vi "Particle Analysis Example.vi"() -> ()   [LabVIEW 2011]
doc: "This example performs a series of grayscale filtering, threshold, binary morphology, and particle analysis operations to measure the areas of all the large circular particles of the image."
uses:
  <vilib>/vision/NI_Vision_Development_Module.lvlib
panel:
  out "Source Image":T1(plugin-control) caption="Rejected Border"
  in  "Font, Size & Style":T2={"Desired Font (Application)"=enum."Application Font", "[User-specified Font]"={"Font Name"="", "Size"=12, "Strikeout?"=FALSE, "Italic?"=FALSE, "Underline?"=FALSE, "Outline?"=FALSE, "Shadow?"=FALSE, "Bold?"=FALSE, "Rotation Angle"=0.0}, "Horizontal Alignment"=0, "Vertical Alignment"=0} {"Vertical Alignment" items=["Bottom", "Top", "Baseline"]; "Horizontal Alignment" items=["Left", "Center", "Right"]; "[User-specified Font]"."Rotation Angle" format="%.2f"}
  in  "Stop":bool
  in  "Run Current Step":bool
  out "Blob Analysis Steps":i32(listbox)
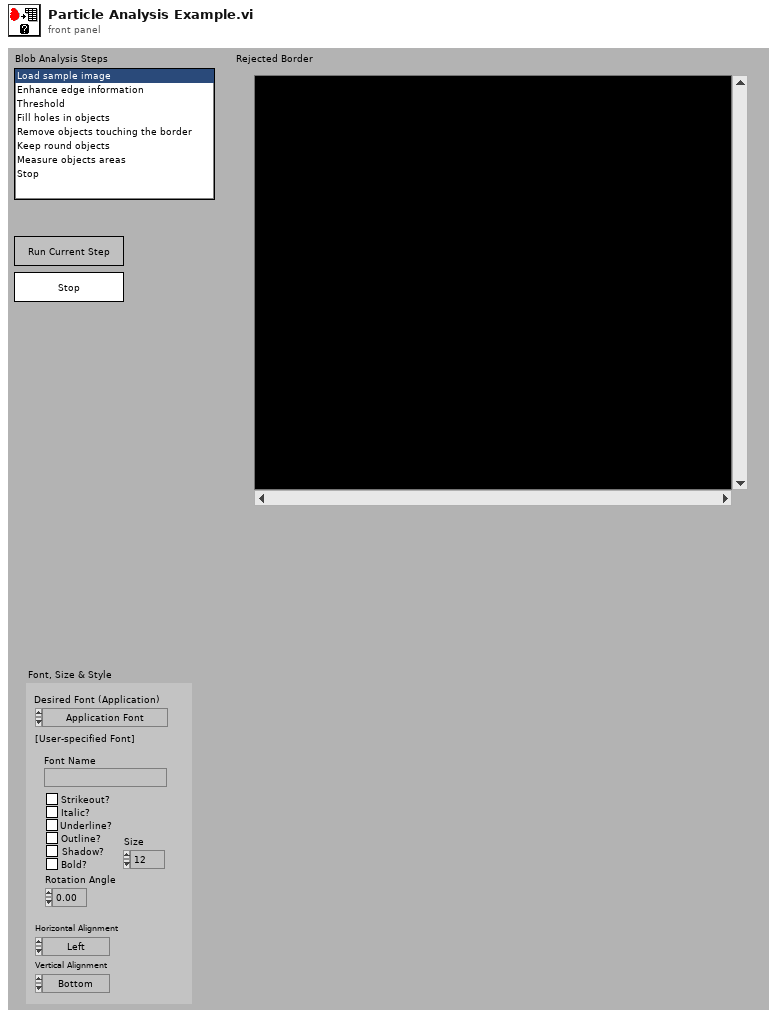
[diagram p1: front panel]
types:
  T1 = typedef "IMAQ Image.ctl" = refnum<image>
  T2 = cluster{"Desired Font (Application)":enum16{"User-specified Font", "Application Font", "System Font", "Dialog Font"}, "[User-specified Font]":cluster{"Font Name":string, "Size":i16, "Strikeout?":bool, "Italic?":bool, "Underline?":bool, "Outline?":bool, "Shadow?":bool, "Bold?":bool, "Rotation Angle":dbl}, "Horizontal Alignment":i16, "Vertical Alignment":i16}
  T3 = enum32{"", "Gradient", "Laplacian", "Smoothing", "Gaussian"}
  T4 = typedef "Particle Parameters" = i32
  T5 = cluster{"Measurement Parameter":T4, "Range Lower Value":dbl, "Range Upper Value":dbl, "Range":bool, "Measurement Type":bool}[]
  T6 = cluster{"Particle Measurements (Pixels)[0]":dbl, "Particle Measurements (Pixels)[1]":dbl, "Particle Measurements (Pixels)[2]":dbl}
  T7 = cluster{"Particle Measurements (Pixels)[0]":dbl, "Particle Measurements (Pixels)[1]":dbl}
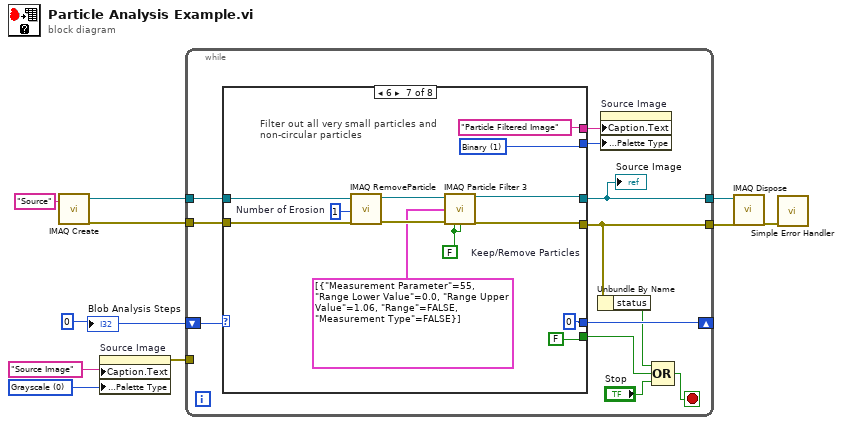
[diagram p0: block diagram]
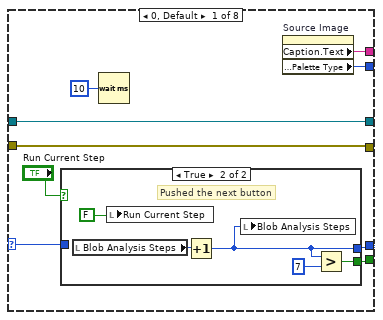
[diagram p2: hidden frame]
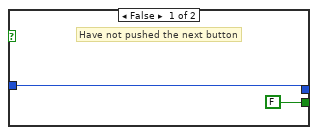
[diagram p3: hidden frame]
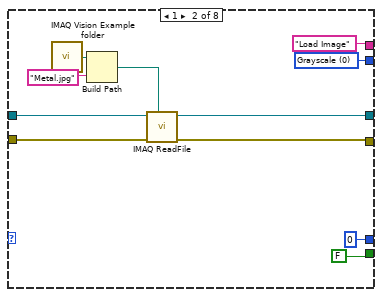
[diagram p4: hidden frame]
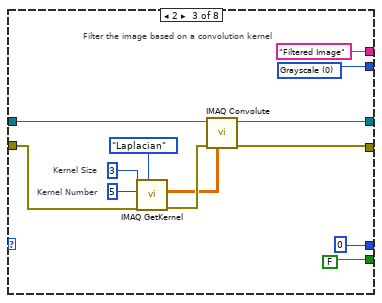
[diagram p5: hidden frame]
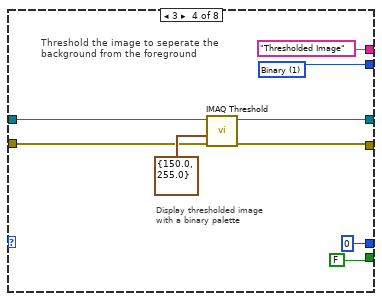
[diagram p6: hidden frame]
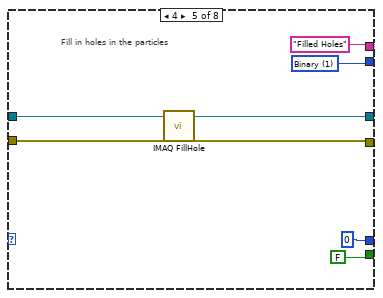
[diagram p7: hidden frame]
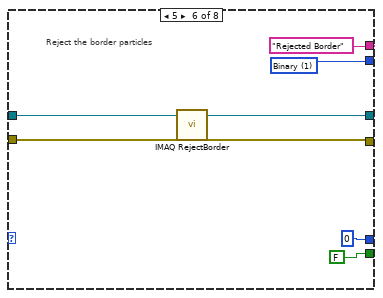
[diagram p8: hidden frame]
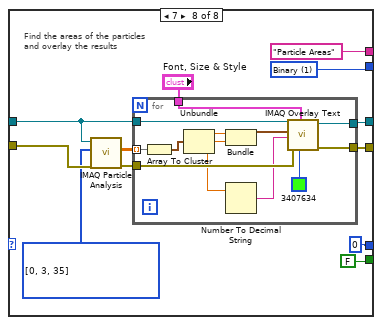
[diagram p9: hidden frame]
diagram:
  w6 = 0
  w7 = u32 0 items=["Grayscale", "Binary", "Gradient", "Rainbow", "Temperature", "User Defined"] ("Palette:Palette Type")
  n1 = call "IMAQ Create"("Image Name"="Source") -> ("New Image"=w2:T1, "error out"=w1:errorcluster)  [unwired: 3 in, 1 out]
  n2 = property on="Source Image" class="ImageControl"("Caption.Text"="Source Image", "Palette:Palette Type"=w7) -> (error out=w9:errorcluster)  [unwired: 2 in, 1 out]
  n3 = while {
    tunnel: w2 -> [w22]
    tunnel: w1 -> [w21]
    shift-right: [w17] -> _
    shift-left: w6 -> [w18]
    tunnel: w9 -> [_]
    tunnel: [w12] -> w5
    tunnel: [w11] -> w4
    stop <- w20 stop-if-true
    n4 = case shown="6" w18 {
      selector: w18 -> [w30 _ _ _ _ _ _ _]
      tunnel: w22 -> [w28 w47 w57 w70 w79 w87 w97 w111]
      tunnel: w21 -> [w29 w46 w51 w63 w73 w81 w91 w103]
      tunnel: [w29 w44 w55 w66 w76 w84 w95 w107] -> w12
      tunnel: [w23 0 0 0 0 0 0 0] -> w17
      tunnel: [w28 w45 w54 w68 w75 w83 w93 w108] -> w11
      tunnel: [w27 "Load Image" ("Title") "Filtered Image" ("Title") "Thresholded Image" ("Title") "Filled Holes" ("Title") "Rejected Border" ("Title") "Particle Filtered Image" ("Title") "Particle Areas" ("Title")] -> w15
      tunnel: [w26 w40 w50 w64 w72 w80 w90 w105] -> w16
      tunnel: [w25 FALSE FALSE FALSE FALSE FALSE FALSE FALSE] -> w13
      frame 0, Default {
        n5 = case shown="True" "Run Current Step" {
          tunnel: w30 -> [w32 _]
          tunnel: [FALSE w35] -> w25
          tunnel: [w32 w34] -> w23
          frame False {
            # "Have not pushed the next button"
          }
          frame True {
            # "Pushed the next button"
            n6 = local read "Blob Analysis Steps"() -> (w37:i32)
            n7 = local write "Run Current Step"(FALSE) -> ()
            n8 = Increment(x=w37) -> (x+1=w34:i32)
            n9 = local write "Blob Analysis Steps"(w34) -> ()
            n10 = Greater?(x=w34, y=7) -> (0:w35:bool)
          }
        }
        n11 = Wait (ms)(milliseconds to wait=u32 10) -> ()  [unwired: 1 out]
        n12 = property on="Source Image" class="ImageControl"() -> ("Caption.Text"=w27:string, "Palette:Palette Type"=w26:u32)  [unwired: 2 in, 2 out]
      }
      frame 1 {
        w40 = u32 0 items=["Grayscale", "Binary", "Gradient", "Rainbow", "Temperature", "User Defined"] ("Palette:Palette Type")
        n13 = call "IMAQ Vision Example folder.vi"() -> ("Example Image Path"=w48:path)  [unwired: 1 out]
        n14 = Build Path(base path=w48, name or relative path="Metal.jpg") -> (appended path=w43:path)
        n15 = call "IMAQ ReadFile"("File Path"=w43, "error in (no error)"=w46, "Image"=w47) -> ("error out"=w44:errorcluster, "Image Out"=w45:T1)  [unwired: 2 in, 5 out]
      }
      frame 2 {
        w50 = u32 0 items=["Grayscale", "Binary", "Gradient", "Rainbow", "Temperature", "User Defined"] ("Palette:Palette Type")
        # "Kernel Number"
        # "Kernel Size"
        # "Filter the image based on a convolution kernel"
        n16 = call "IMAQ GetKernel"("Kernel Family"=T3."Laplacian", "error in (no error)"=w51, "Kernel Number"=5, "Kernel Size (3,5,...)"=3) -> ("error out"=w62:errorcluster, "Kernel"=w61:sgl[][])  [unwired: 1 in, 5 out]
        n17 = call "IMAQ Convolute"("Kernel"=w61, "error in (no error)"=w62, "Image Src"=w57) -> ("error out"=w55:errorcluster, "Image Dst Out"=w54:T1)  [unwired: 4 in, 3 out]
      }
      frame 3 {
        w64 = u32 1 items=["Grayscale", "Binary", "Gradient", "Rainbow", "Temperature", "User Defined"] ("Palette:Palette Type")
        # "Display thresholded image with a binary palette"
        # "Threshold the image to seperate the background from the foreground"
        n18 = call "IMAQ Threshold"("error in (no error)"=w63, "Range"=cluster{"Lower value":sgl, "Upper value":sgl} {"Lower value"=150.0, "Upper value"=255.0}, "Image Src"=w70) -> ("error out"=w66:errorcluster, "Image Dst Out"=w68:T1)  [unwired: 3 in, 4 out]
      }
      frame 4 {
        w72 = u32 1 items=["Grayscale", "Binary", "Gradient", "Rainbow", "Temperature", "User Defined"] ("Palette:Palette Type")
        # "Fill in holes in the particles"
        n19 = call "IMAQ FillHole"("error in (no error)"=w73, "Image Src"=w79) -> ("error out"=w76:errorcluster, "Image Dst Out"=w75:T1)  [unwired: 2 in, 2 out]
      }
      frame 5 {
        w80 = u32 1 items=["Grayscale", "Binary", "Gradient", "Rainbow", "Temperature", "User Defined"] ("Palette:Palette Type")
        # "Reject the border particles"
        n20 = call "IMAQ RejectBorder"("error in (no error)"=w81, "Image Src"=w87) -> ("error out"=w84:errorcluster, "Image Dst Out"=w83:T1)  [unwired: 2 in, 2 out]
      }
      frame 6 {
        w90 = u32 1 items=["Grayscale", "Binary", "Gradient", "Rainbow", "Temperature", "User Defined"] ("Palette:Palette Type")
        w98 = 1  # Number of Erosion
        w88 = FALSE  # Keep/Remove Particles
        # "Filter out all very small particles and non-circular particles"
        n21 = call "IMAQ RemoveParticle"("error in (no error)"=w91, "Number of Erosion"=w98, "Image Src"=w97) -> ("error out"=w100:errorcluster, "Image Dst Out"=w99:T1)  [unwired: 4 in, 3 out]
        n22 = call "IMAQ Particle Filter 3"("Image Src"=w99, "Selection Values"=T5 [{"Measurement Parameter"=55, "Range Lower Value"=0.0, "Range Upper Value"=1.06, "Range"=FALSE, "Measurement Type"=FALSE}], "Keep/Remove Particles (F)"=w88, "error in (no error)"=w100, "Fill Holes? (F)"=w88) -> ("Image Dst Out"=w93:T1, "error out"=w95:errorcluster)  [unwired: 4 in, 5 out]
      }
      frame 7 {
        w102 = T4[] [0, 3, 35] items=["Center of Mass X", "Center of Mass Y", "First Pixel X", "First Pixel Y", "Bounding Rect Left", "Bounding Rect Top", "Bounding Rect Right", "Bounding Rect Bottom", "Max Feret Diameter Start X", "Max Feret Diameter Start Y", "Max Feret Diameter End X", "Max Feret Diameter End Y", "Max Horiz. Segment Length Left", "Max Horiz. Segment Length Right", "Max Horiz. Segment Length Row", "-", "Bounding Rect Width", "Bounding Rect Height", "Bounding Rect Diagonal", "Perimeter", "Convex Hull Perimeter", "Holes' Perimeter", "Max Feret Diameter", "Equivalent Ellipse Major Axis", "Equivalent Ellipse Minor Axis", "Equivalent Ellipse Minor Axis (Feret)", "Equivalent Rect Long Side", "Equivalent Rect Short Side", "Equivalent Rect Diagonal", "Equivalent Rect Short Side (Feret)", "Average Horiz. Segment Length", "Average Vert. Segment Length", "Hydraulic Radius", "Waddel Disk Diameter", "-", "Area", "Holes' Area", "Particle & Holes' Area", "Convex Hull Area", "Image Area", "-", "Number of Holes", "Number of Horiz. Segments", "Number of Vert. Segments", "-", "Orientation", "Max Feret Diameter Orientation", "-", "% Area/Image Area", "% Area/(Particle & Holes' Area)", "Ratio of Equivalent Ellipse Axes", "Ratio of Equivalent Rect Sides", "-", "Elongation Factor", "Compactness Factor", "Heywood Circularity Factor", "Type Factor", "-", "Sum X", "Sum Y", "Sum XX", "Sum XY", "Sum YY", "Sum XXX", "Sum XXY", "Sum XYY", "Sum YYY", "-", "Moment of Inertia XX", "Moment of Inertia XY", "Moment of Inertia YY", "Moment of Inertia XXX", "Moment of Inertia XXY", "Moment of Inertia XYY", "Moment of Inertia YYY", "Norm. Moment of Inertia XX", "Norm. Moment of Inertia XY", "Norm. Moment of Inertia YY", "Norm. Moment of Inertia XXX", "Norm. Moment of Inertia XXY", "Norm. Moment of Inertia XYY", "Norm. Moment of Inertia YYY", "Hu Moment 1", "Hu Moment 2", "Hu Moment 3", "Hu Moment 4", "Hu Moment 5", "Hu Moment 6", "Hu Moment 7"] ("Pixel Measurements")
        w105 = u32 1 items=["Grayscale", "Binary", "Gradient", "Rainbow", "Temperature", "User Defined"] ("Palette:Palette Type")
        # "Find the areas of the particles and overlay the results"
        n23 = call "IMAQ Particle Analysis"("error in (no error)"=w103, "Pixel Measurements"=w102, "Image"=w111) -> ("error out"=w112:errorcluster, "Particle Measurements (Pixels)"=w101:dbl[][])  [unwired: 2 in, 5 out]
        n24 = for {
          tunnel: w112 -> [w125]
          tunnel: [w124] -> w107
          tunnel: [w123] -> w108
          tunnel: w111 -> [w120]
          tunnel: "Font, Size & Style" -> [w114]
          tunnel: w101 -> [w113] mode=indexing
          n25 = Array To Cluster(array=w113) -> (cluster=w119:T6)
          n26 = Unbundle(w119) -> ("Particle Measurements (Pixels)[0]"=w118:dbl, "Particle Measurements (Pixels)[1]"=w117:dbl, "Particle Measurements (Pixels)[2]"=w115:dbl)
          n27 = Bundle("Particle Measurements (Pixels)[0]"=w118, "Particle Measurements (Pixels)[1]"=w117) -> (w116:T7)  [unwired: 1 out]
          n28 = Number To Decimal String(number=w115) -> (decimal integer string=w122:string)  [unwired: 1 out]
          n29 = call "IMAQ Overlay Text"("Text Color (black)"=u32 3407634, "Font, Size & Style"=w114, "error in (no error)"=w125, "String"=w122, "Origin"=w116, "Image"=w120) -> ("error out"=w124:errorcluster, "Image Out"=w123:T1)  [unwired: 2 in, 2 out]
        }
      }
    }
    "Source Image" <- w11
    n30 = Unbundle By Name(w12) -> ("status"=w14:bool)
    n31 = property on="Source Image" class="ImageControl"("Caption.Text"=w15, "Palette:Palette Type"=w16) -> ()  [unwired: 2 in, 2 out]
    n32 = Compound Arithmetic op=OR(w14, w13, "Stop") -> (w20:bool)
  }
  n33 = call "IMAQ Dispose"("Image"=w4, "error in (no error)"=w5) -> ("error out"=w3:errorcluster)  [unwired: 1 in, 3 out]
  n34 = call <vilib>:"Simple Error Handler.vi"("error in (no error)"=w3) -> ()  [unwired: 1 in, 8 out]
  "Blob Analysis Steps" <- w6
